vi "HitrapGUI.HTLE_TR6BT1-copy.vi"() -> ()   [LabVIEW 2014, in "HT_CSGUI.lvlib"]
uses:
  HT_CSGUI.lvlib
  CSlibraries/UtilityLib/UtilityLib.lvlib
  CSCore/CSSystem/CSSystemLib/CSSystemLib.lvlib
  CSlibraries/GUILib/GUILib.lvlib
  CSlibraries/UtilityLib/UtilityLib.valueStatus.ctl
  CSCore/CSSystem/CoreDefs/CoreDefs.rawDataType.ctl
  CSCore/CSSystem/CoreLib/CoreLib.lvlib
  CSCore/CSSystem/CoreLib/CoreLib.double 2 byte array.vi
  CSlibraries/GUILib/GUILib.userEventsMainType.ctl
  lib.lib/DimLVEvent/DimIndicators/DimIndicators.anyType.ctl
  CSlibraries/GUILib/GUILib.simpleNumeric.ctl
  CSlibraries/GUILib/GUILib.basicNumeric.ctl
panel:
  in  "showHigh":bool=TRUE
  in  "TR6BT1Trap17_H":bool=TRUE
  in  "TR6BT1Trap16_H":bool=TRUE
  in  "TR6BT1Trap15_H":bool=TRUE
  in  "TR6BT1Trap14_H":bool=TRUE
  in  "TR6BT1Trap13_H":bool=TRUE
  in  "TR6BT1Trap12_H":bool=TRUE
  in  "TR6BT1Trap8_H":bool=TRUE
  in  "TR6BT1Trap7_H":bool=TRUE
  in  "TR6BT1Trap5_H":bool=TRUE
  in  "TR6BT1Trap4_H":bool=TRUE
  in  "TR6BT1Trap3_H":bool=TRUE
  in  "TR6BT1Trap2_H":bool=TRUE
  in  "TR6BT1Trap21_H":bool=TRUE
  in  "TR6BT1Trap20_H":bool=TRUE
  in  "TR6BT1Trap19_H":bool=TRUE
  in  "TR6BT1Trap18_H":bool=TRUE
  in  "TR6BT1Trap11_H":bool=TRUE
  in  "TR6BT1Trap10_H":bool=TRUE
  in  "TR6BT1Trap9_H":bool=TRUE
  in  "TR6BT1Trap6_H":bool=TRUE
  in  "TR6BT1Trap1_H":bool=TRUE
  in  "TR6BT1Trap2":bool=TRUE
  in  "TR6BT1Trap21":bool=TRUE
  in  "TR6BT1Trap20":bool=TRUE
  in  "TR6BT1Trap19":bool=TRUE
  in  "TR6BT1Trap18":bool=TRUE
  in  "TR6BT1Trap17":bool=TRUE
  in  "TR6BT1Trap16":bool=TRUE
  in  "TR6BT1Trap15":bool=TRUE
  in  "TR6BT1Trap14":bool=TRUE
  in  "TR6BT1Trap13":bool=TRUE
  in  "TR6BT1Trap12":bool=TRUE
  in  "TR6BT1Trap11":bool=TRUE
  in  "TR6BT1Trap10":bool=TRUE
  in  "TR6BT1Trap9":bool=TRUE
  in  "TR6BT1Trap8":bool=TRUE
  in  "TR6BT1Trap7":bool=TRUE
  in  "TR6BT1Trap6":bool=TRUE
  in  "TR6BT1Trap5":bool=TRUE
  in  "TR6BT1Trap4":bool=TRUE
  in  "TR6BT1Trap3":bool=TRUE
  in  "TR6BT1Trap11_HCtl":T1 {"nom" step=1.0}
  in  "TR6BT1Trap11Ctl":T1 {"nom" step=1.0}
  in  "TR6BT1Trap10Ctl":T1 {"nom" step=1.0}
  in  "TR6BT1Trap10_HCtl":T1 {"nom" step=1.0}
  in  "TR6BT1Trap9Ctl":T1 {"nom" step=1.0}
  in  "TR6BT1Trap4_HCtl":T1 {"nom" step=1.0}
  in  "TR6BT1Trap9_HCtl":T1 {"nom" step=1.0}
  in  "TR6BT1Trap12_HCtl":T1 {"nom" step=1.0}
  in  "TR6BT1Trap21_HCtl":T1 {"nom" step=1.0}
  in  "TR6BT1Trap8_HCtl":T1 {"nom" step=1.0}
  in  "TR6BT1Trap7_HCtl":T1 {"nom" step=1.0}
  in  "TR6BT1Trap7Ctl":T1 {"nom" step=1.0}
  in  "TR6BT1Trap5Ctl":T1 {"nom" step=1.0}
  in  "TR6BT1Trap12Ctl":T1 {"nom" step=1.0}
  in  "TR6BT1Trap21Ctl":T1 {"nom" step=1.0}
  in  "TR6BT1Trap8Ctl":T1 {"nom" step=1.0}
  in  "TR6BT1Trap6Ctl":T1 {"nom" step=1.0}
  in  "TR6BT1Trap6_HCtl":T1 {"nom" step=1.0}
  in  "TR6BT1Trap5_HCtl":T1 {"nom" step=1.0}
  in  "TR6BT1Trap4Ctl":T1 {"nom" step=1.0}
  in  "TR6BT1Trap3_HCtl":T1 {"nom" step=1.0}
  in  "TR6BT1Trap2Ctl":T1 {"nom" step=1.0}
  in  "TR6BT1Trap3Ctl":T1 {"nom" step=1.0}
  in  "TR6BT1Trap2_HCtl":T1 {"nom" step=1.0}
  in  "TR6BT1Trap19Ctl":T1 {"nom" step=1.0}
  in  "TR6BT1Trap20_HCtl":T1 {"nom" step=1.0}
  in  "TR6BT1Trap17_HCtl":T1 {"nom" step=1.0}
  in  "TR6BT1Trap18_HCtl":T1 {"nom" step=1.0}
  in  "TR6BT1Trap20Ctl":T1 {"nom" step=1.0}
  in  "TR6BT1Trap19_HCtl":T1 {"nom" step=1.0}
  in  "TR6BT1Trap18Ctl":T1 {"nom" step=1.0}
  in  "TR6BT1Trap17Ctl":T1 {"nom" step=1.0}
  in  "TR6BT1Trap16Ctl":T1 {"nom" step=1.0}
  in  "TR6BT1Trap15Ctl":T1 {"nom" step=1.0}
  in  "TR6BT1Trap16_HCtl":T1 {"nom" step=1.0}
  in  "TR6BT1Trap15_HCtl":T1 {"nom" step=1.0}
  in  "TR6BT1Trap14Ctl":T1 {"nom" step=1.0}
  in  "TR6BT1Trap14_HCtl":T1 {"nom" step=1.0}
  in  "TR6BT1Trap13Ctl":T1 {"nom" step=1.0}
  in  "TR6BT1Trap13_HCtl":T1 {"nom" step=1.0}
  in  "TR6BT1Trap1_HCtl":T1 {"nom" step=1.0}
  in  "OK Button":bool
  in  "TR6BT1Trap1Ctl":T1 {"nom" step=1.0}
  in  "TR6BT1Trap1":bool=TRUE
  in  "analog1Ctl":T1 {"nom" step=1.0}
  in  "analog1":bool=TRUE
  out "subSystem1State":string
  in  "subSystem1":bool
  out "subSystem1StateQuality":string
  in  "subControllersIgnoredDIM":T3
  in  "iniData":string
  in  "stop":bool
  in  "dummy":bool
  in  "parentSystem":bool
  in  "userEvent":refnum<user-event>
  # "TR6BT1"
  # "1"
  # "2"
  # "3"
  # "4"
  # "5"
  # "6"
  # "7"
  # "8"
  # "9"
  # "10"
  # "11"
  # "12"
  # "13"
  # "14"
  # "15"
  # "16"
  # "17"
  # "18"
  # "19"
  # "20"
  # "21"
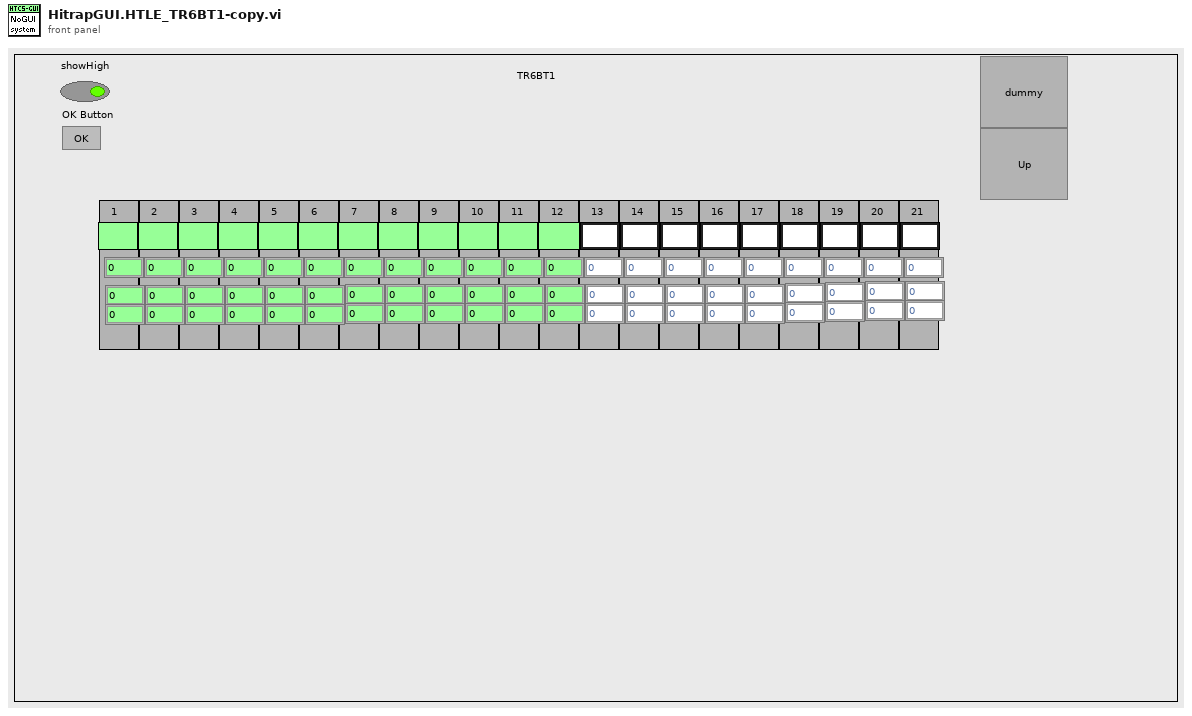
[diagram p1: front panel]
types:
  T1 = typedef "GUILib.lvlib/GUILib.simpleNumeric.ctl" = cluster{"nom":T2, "act":dbl, "inc":dbl}
  T2 = typedef "GUILib.lvlib/GUILib.basicNumeric.ctl" = dbl
  T3 = typedef "DimIndicators.lvlib/DimIndicators.anyType.ctl" = cluster{"data":string, "no link":bool, "quality":i32, "timeStamp":dbl}
  T4 = typedef "UtilityLib.lvlib/UtilityLib.valueStatus.ctl" = enum16{"no info available", "stand by/off", "on", "warning", "alarm/malfunction", "not implemented", "user action required", "important information", "system default", "control default", "indicator default", "button default"}
  T5 = typedef "CoreDefs.rawDataType.ctl" = i8[]
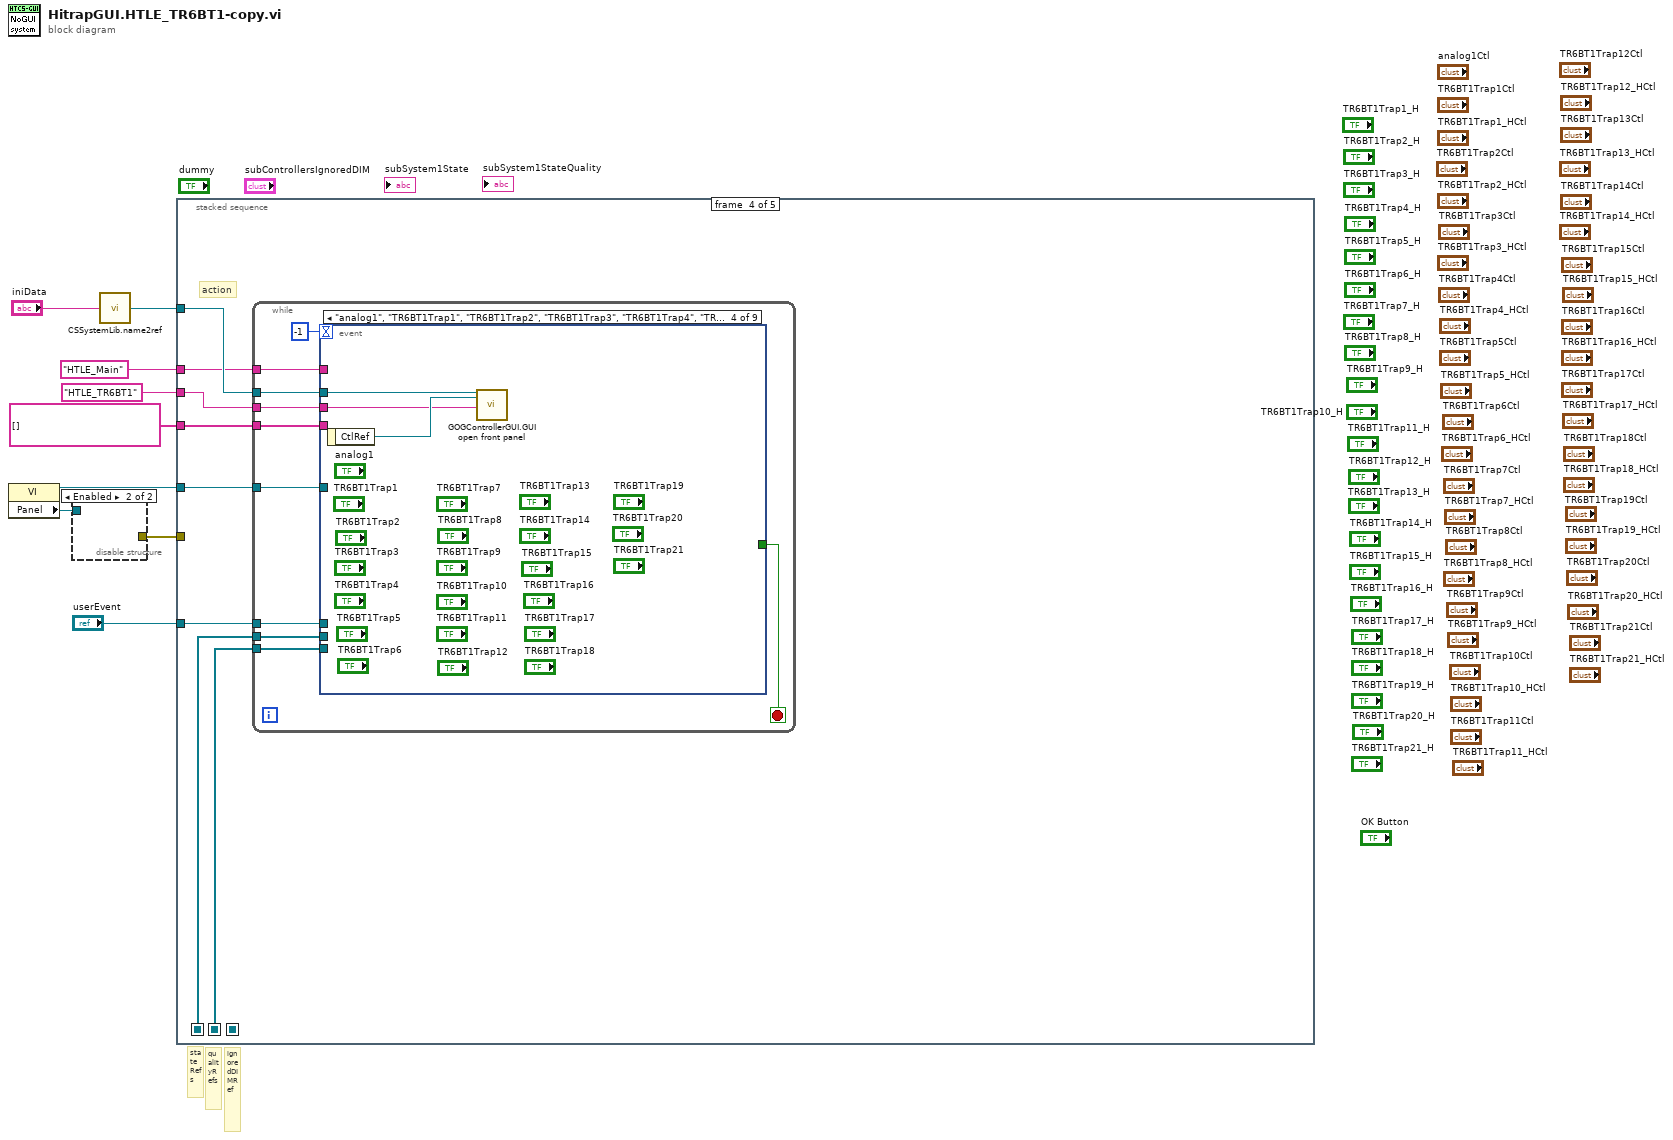
[diagram p0: block diagram]
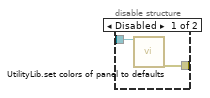
[diagram p2: hidden frame]
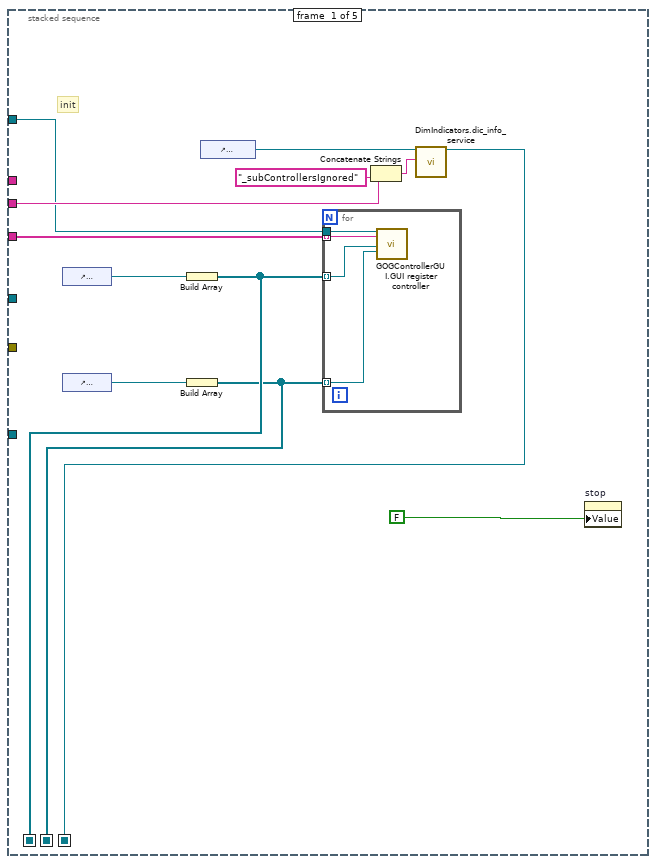
[diagram p3: hidden frame]
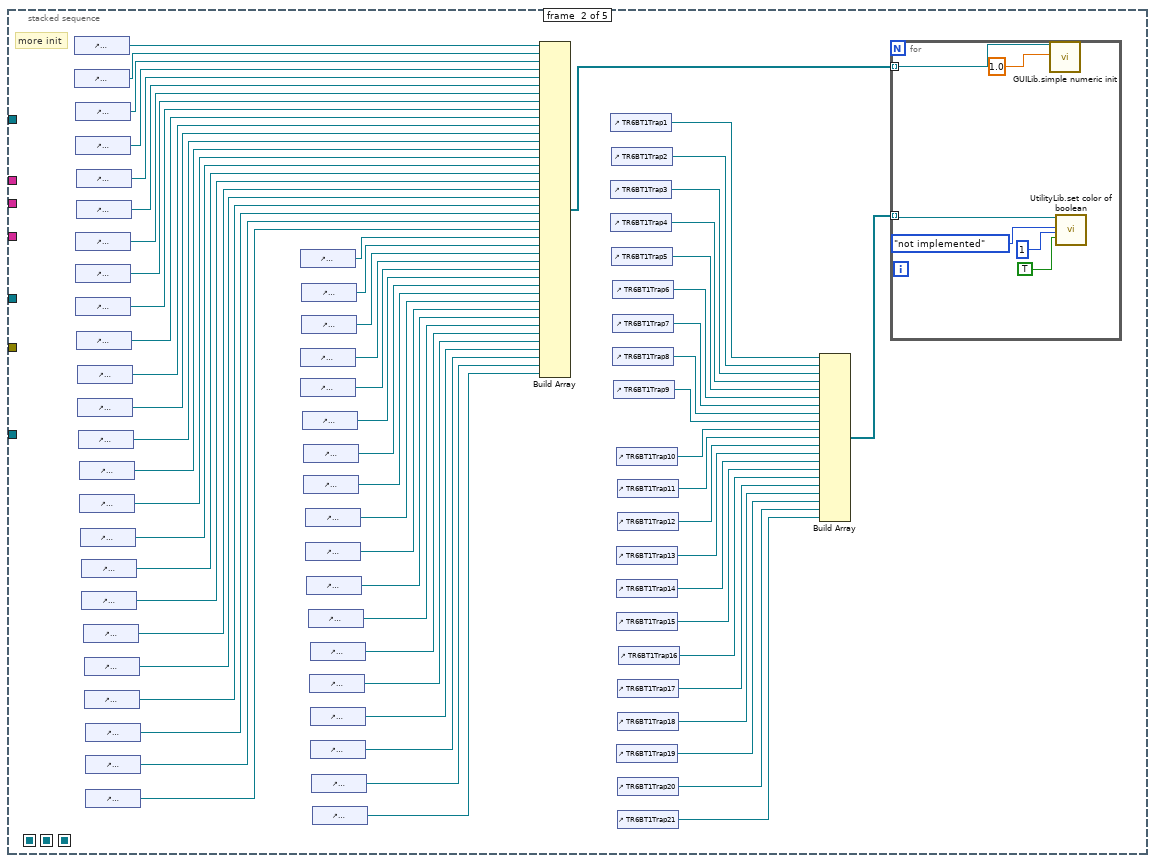
[diagram p4: hidden frame]
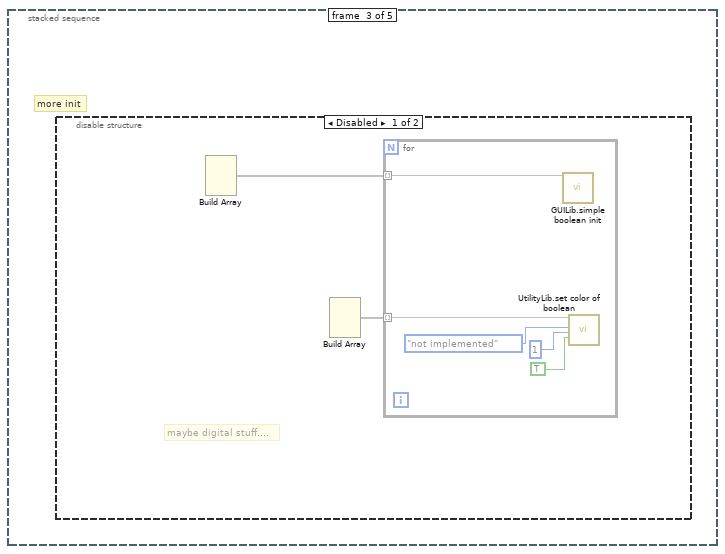
[diagram p5: hidden frame]
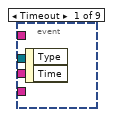
[diagram p7: hidden frame]
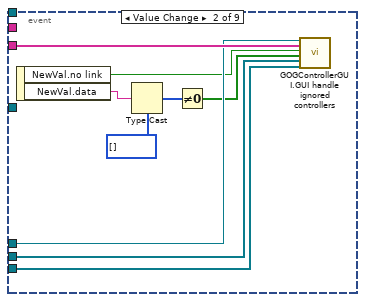
[diagram p8: hidden frame]
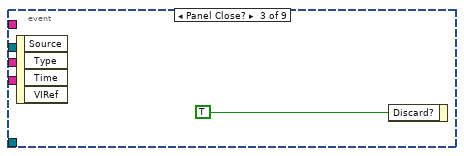
[diagram p9: hidden frame]
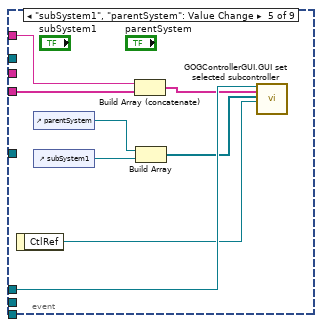
[diagram p10: hidden frame]
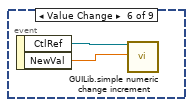
[diagram p11: hidden frame]
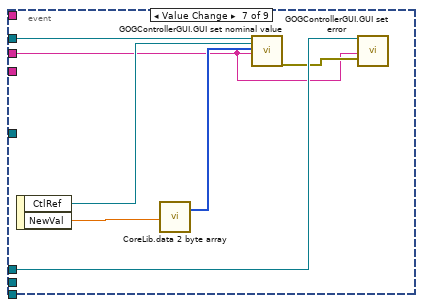
[diagram p12: hidden frame]
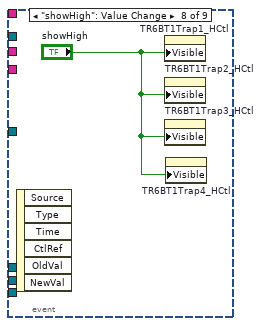
[diagram p13: hidden frame]
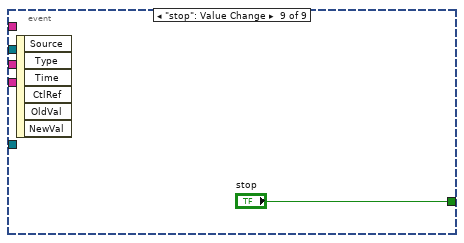
[diagram p14: hidden frame]
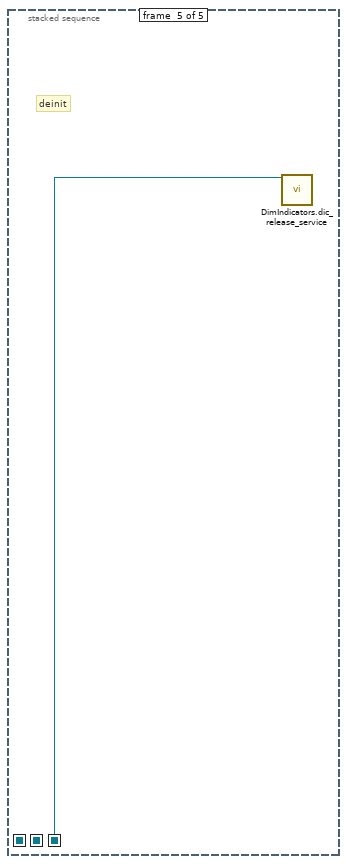
[diagram p15: hidden frame]
diagram:
  # "qualityRefs"
  # "ignoredDIMRef"
  # "stateRefs"
  n1 = property class="VI"() -> (reference out=w7:refnum<vi>, "Panel"=w8:refnum<vi>)  [unwired: 2 in, 1 out]
  n2 = disable-structure shown="Enabled" {
    disable-tunnel: w8 -> [w11 _]
    disable-tunnel: [w10 _] -> w6
    frame Disabled {
      n3 = call "UtilityLib.set colors of panel to defaults.vi"("Front Panel"=w11) -> ("error out"=w10:errorcluster)  [unwired: 18 in]
    }
    frame Enabled {
    }
  }
  n4 = call "CSSystemLib.name2ref.vi"("name"="iniData") -> ("obj refnum"=w2:refnum<vi>)
  n5 = stacked-sequence {
    seq-local: [w13 _ _ _ _] -> [_ _ _ _ w166]
    seq-local: [w14 _ _ _ _] -> [_ _ _ w120 _]
    seq-local: [w12 _ _ _ _] -> [_ _ _ w119 _]
    tunnel: "userEvent" -> [_ _ _ w123 _]
    tunnel: w7 -> [_ _ _ w122 _]
    tunnel: w6 -> [_ _ _ _ _]
    tunnel: "HTLE_TR6BT1" -> [w19 _ _ w117 _]
    tunnel: string[] [] -> [w18 _ _ w121 _]
    tunnel: w2 -> [w17 _ _ w118 _]
    tunnel: "HTLE_Main" -> [_ _ _ w116 _]
    frame #0 {
      # "init"
      n6 = control-ref of="dummySubSystemState"() -> (w16:refnum<vi>)
      n7 = control-ref of="dummySubSystemStateQuality"() -> (w15:refnum<vi>)
      n8 = Build Array(w16) -> (w14:refnum<vi>[])
      n9 = Build Array(w15) -> (w12:refnum<vi>[])
      n10 = control-ref of="subControllersIgnoredDIM"() -> (w20:refnum<vi>)
      n11 = for {
        tunnel: w14 -> [w27] mode=indexing
        tunnel: w18 -> [w25] mode=indexing
        tunnel: w12 -> [w24] mode=indexing
        tunnel: w17 -> [w26]
        n12 = call "GOGControllerGUI.GUI register controller.vi"("i ref in"=w26, "controllerName"=w25, "subSystemState"=w27, "subSystemStateQuality"=w24) -> ()  [unwired: 14 in, 2 out]
      }
      n13 = Concatenate Strings(w19, "_subControllersIgnored" ("string")) -> (w22:string)
      n14 = call "DimIndicators.dic_info_service.vi"("controlRef"=w20, "serviceName"=w22) -> ("controlRef out"=w13:refnum<vi>)  [unwired: 16 in, 1 out]
      n15 = property on="stop" class="Bool (strict)"("Value"=FALSE ("stop")) -> ()  [unwired: 2 in, 2 out]
    }
    frame #1 {
      # "more init"
      n16 = control-ref of="TR6BT1Trap1Ctl"() -> (w92:refnum<vi>)
      n17 = control-ref of="TR6BT1Trap1_HCtl"() -> (w88:refnum<vi>)
      n18 = control-ref of="TR6BT1Trap2Ctl"() -> (w87:refnum<vi>)
      n19 = control-ref of="TR6BT1Trap2_HCtl"() -> (w86:refnum<vi>)
      n20 = control-ref of="TR6BT1Trap4Ctl"() -> (w83:refnum<vi>)
      n21 = control-ref of="TR6BT1Trap4_HCtl"() -> (w82:refnum<vi>)
      n22 = control-ref of="TR6BT1Trap5Ctl"() -> (w81:refnum<vi>)
      n23 = control-ref of="TR6BT1Trap3Ctl"() -> (w85:refnum<vi>)
      n24 = control-ref of="TR6BT1Trap3_HCtl"() -> (w84:refnum<vi>)
      n25 = control-ref of="TR6BT1Trap5_HCtl"() -> (w80:refnum<vi>)
      n26 = control-ref of="TR6BT1Trap6Ctl"() -> (w79:refnum<vi>)
      n27 = control-ref of="TR6BT1Trap6_HCtl"() -> (w78:refnum<vi>)
      n28 = control-ref of="TR6BT1Trap7Ctl"() -> (w77:refnum<vi>)
      n29 = control-ref of="TR6BT1Trap7_HCtl"() -> (w76:refnum<vi>)
      n30 = control-ref of="TR6BT1Trap8Ctl"() -> (w75:refnum<vi>)
      n31 = control-ref of="TR6BT1Trap8_HCtl"() -> (w74:refnum<vi>)
      n32 = control-ref of="TR6BT1Trap9Ctl"() -> (w73:refnum<vi>)
      n33 = control-ref of="TR6BT1Trap9_HCtl"() -> (w72:refnum<vi>)
      n34 = control-ref of="TR6BT1Trap10Ctl"() -> (w70:refnum<vi>)
      n35 = control-ref of="TR6BT1Trap10_HCtl"() -> (w69:refnum<vi>)
      n36 = control-ref of="TR6BT1Trap11Ctl"() -> (w68:refnum<vi>)
      n37 = control-ref of="TR6BT1Trap11_HCtl"() -> (w67:refnum<vi>)
      n38 = control-ref of="TR6BT1Trap12Ctl"() -> (w66:refnum<vi>)
      n39 = control-ref of="TR6BT1Trap12_HCtl"() -> (w65:refnum<vi>)
      n40 = control-ref of="TR6BT1Trap13Ctl"() -> (w64:refnum<vi>)
      n41 = control-ref of="TR6BT1Trap14_HCtl"() -> (w61:refnum<vi>)
      n42 = control-ref of="TR6BT1Trap15Ctl"() -> (w60:refnum<vi>)
      n43 = control-ref of="TR6BT1Trap13_HCtl"() -> (w63:refnum<vi>)
      n44 = control-ref of="TR6BT1Trap14Ctl"() -> (w62:refnum<vi>)
      n45 = control-ref of="TR6BT1Trap15_HCtl"() -> (w59:refnum<vi>)
      n46 = control-ref of="TR6BT1Trap16Ctl"() -> (w58:refnum<vi>)
      n47 = control-ref of="TR6BT1Trap16_HCtl"() -> (w57:refnum<vi>)
      n48 = control-ref of="TR6BT1Trap17Ctl"() -> (w56:refnum<vi>)
      n49 = control-ref of="TR6BT1Trap17_HCtl"() -> (w55:refnum<vi>)
      n50 = control-ref of="TR6BT1Trap18Ctl"() -> (w54:refnum<vi>)
      n51 = control-ref of="TR6BT1Trap18_HCtl"() -> (w53:refnum<vi>)
      n52 = control-ref of="TR6BT1Trap19_HCtl"() -> (w51:refnum<vi>)
      n53 = control-ref of="TR6BT1Trap19Ctl"() -> (w52:refnum<vi>)
      n54 = control-ref of="TR6BT1Trap20Ctl"() -> (w50:refnum<vi>)
      n55 = control-ref of="TR6BT1Trap20_HCtl"() -> (w49:refnum<vi>)
      n56 = control-ref of="TR6BT1Trap21Ctl"() -> (w48:refnum<vi>)
      n57 = control-ref of="TR6BT1Trap21_HCtl"() -> (w47:refnum<vi>)
      n58 = Build Array(w92, w88, w87, w86, w85, w84, w83, w82, w81, w80, w79, w78, w77, w76, w75, w74, w73, w72, w70, w69, w68, w67, w66, w65, w64, w63, w62, w61, w60, w59, w58, w57, w56, w55, w54, w53, w52, w51, w50, w49, w48, w47) -> (w91:refnum<vi>[])
      n59 = control-ref of="TR6BT1Trap1"() -> (w90:refnum<vi>)
      n60 = control-ref of="TR6BT1Trap3"() -> (w46:refnum<vi>)
      n61 = control-ref of="TR6BT1Trap4"() -> (w45:refnum<vi>)
      n62 = control-ref of="TR6BT1Trap2"() -> (w71:refnum<vi>)
      n63 = control-ref of="TR6BT1Trap5"() -> (w44:refnum<vi>)
      n64 = control-ref of="TR6BT1Trap6"() -> (w43:refnum<vi>)
      n65 = control-ref of="TR6BT1Trap7"() -> (w42:refnum<vi>)
      n66 = control-ref of="TR6BT1Trap8"() -> (w41:refnum<vi>)
      n67 = control-ref of="TR6BT1Trap9"() -> (w40:refnum<vi>)
      n68 = control-ref of="TR6BT1Trap10"() -> (w39:refnum<vi>)
      n69 = control-ref of="TR6BT1Trap13"() -> (w36:refnum<vi>)
      n70 = control-ref of="TR6BT1Trap14"() -> (w35:refnum<vi>)
      n71 = control-ref of="TR6BT1Trap15"() -> (w34:refnum<vi>)
      n72 = control-ref of="TR6BT1Trap19"() -> (w30:refnum<vi>)
      n73 = control-ref of="TR6BT1Trap11"() -> (w38:refnum<vi>)
      n74 = control-ref of="TR6BT1Trap12"() -> (w37:refnum<vi>)
      n75 = control-ref of="TR6BT1Trap17"() -> (w32:refnum<vi>)
      n76 = control-ref of="TR6BT1Trap18"() -> (w31:refnum<vi>)
      n77 = control-ref of="TR6BT1Trap20"() -> (w29:refnum<vi>)
      n78 = control-ref of="TR6BT1Trap21"() -> (w28:refnum<vi>)
      n79 = control-ref of="TR6BT1Trap16"() -> (w33:refnum<vi>)
      n80 = Build Array(w90, w71, w46, w45, w44, w43, w42, w41, w40, w39, w38, w37, w36, w35, w34, w33, w32, w31, w30, w29, w28) -> (w89:refnum<vi>[])
      n81 = for {
        tunnel: w91 -> [w98] mode=indexing
        tunnel: w89 -> [w94] mode=indexing
        n82 = call "GUILib.simple numeric init.vi"("ctlRef"=w98, "increment"=1.0) -> ()  [unwired: 16 in, 2 out]
        n83 = call "UtilityLib.set color of boolean.vi"("button"=w94, "valueStatus"=UtilityLib.valueStatus."not implemented", "nOfPair (0)"=1, "setTRUEColor (FALSE)"=TRUE) -> ()  [unwired: 15 in, 1 out]
      }
    }
    frame #2 {
      # "more init"
      n84 = disable-structure shown="Disabled" {
        frame Disabled {
          # "maybe digital stuff...."
          n85 = Build Array() -> (w105:void[], w110:dbl, w109:dbl, w108:dbl, w107:dbl, w106:dbl)
          n86 = Build Array() -> (w99:void[], w104:dbl, w103:dbl, w102:dbl, w101:dbl, w100:dbl)
          n87 = for {
            tunnel: w105 -> [w115] mode=indexing
            tunnel: w99 -> [w111] mode=indexing
            n88 = call "GUILib.simple boolean init.vi"("ctlRef"=w115) -> ()  [unwired: 17 in, 2 out]
            n89 = call "UtilityLib.set color of boolean.vi"("button"=w111, "valueStatus"=UtilityLib.valueStatus."not implemented", "nOfPair (0)"=1, "setTRUEColor (FALSE)"=TRUE) -> ()  [unwired: 15 in, 1 out]
          }
        }
        frame Enabled {
        }
      }
    }
    frame #3 {
      # "action"
      n90 = while {
        tunnel: w123 -> [w133]
        tunnel: w122 -> [w131]
        tunnel: w121 -> [w129]
        tunnel: w120 -> [w128]
        tunnel: w119 -> [w127]
        tunnel: w118 -> [w126]
        tunnel: w117 -> [w125]
        tunnel: w116 -> [w124]
        stop <- w130 stop-if-true
        n91 = event shown="[3] \"analog1\", \"TR6BT1Trap1\", \"TR6BT1Trap2\", \"TR6BT1Trap3\", \"TR6BT1Trap4\", \"TR6BT1Trap5\", \"TR6BT1Trap6\", \"TR6BT1Trap7\", \"TR6BT1Trap8\", \"TR6BT1Trap9\", \"TR6BT1Trap10\", \"TR6BT1Trap11\", \"TR6BT1Trap12\", \"TR6BT1Trap13\", \"TR6BT1Trap14\", \"TR6BT1Trap15\", \"TR6BT1Trap16\", \"TR6BT1Trap17\", \"TR6BT1Trap18\", \"TR6BT1Trap19\", \"TR6BT1Trap20\", \"TR6BT1Trap21\": Value Change" {
          selector: _ -> [_ _ _ _ _ _ _ _ _]
          dyn-events: _ -> [_ _ _ _ _ _ _ _ _]
          timeout: -1 -> [_ _ _ _ _ _ _ _ _]
          tunnel: w133 -> [_ w138 _ _ w153 _ w159 _ _]
          tunnel: w131 -> [_ _ _ _ _ _ _ _ _]
          tunnel: [_ _ _ _ _ _ _ _ "stop"] -> w130
          tunnel: w129 -> [_ w139 _ _ w149 _ _ _ _]
          tunnel: w128 -> [_ w135 _ _ _ _ _ _ _]
          tunnel: w127 -> [_ w134 _ _ _ _ _ _ _]
          tunnel: w126 -> [_ _ _ w146 _ _ w163 _ _]
          tunnel: w125 -> [_ _ _ w144 _ _ w157 _ _]
          tunnel: w124 -> [_ _ _ _ w148 _ _ _ _]
          event Timeout {
            n92 = event-data() -> ()  [unwired: 1 in, 2 out]
          }
          event Value Change {
            n93 = event-data() -> ("NewVal.no link"=w137:bool, "NewVal.data"=w140:string)  [unwired: 1 in]
            n94 = Type Cast(type=T5 [] ("Array"), x=w140) -> (*(type *) &x=w142:T5)
            n95 = Not Equal To 0?(x=w142) -> (x != 0?=w136:bool[])
            n96 = call "GOGControllerGUI.GUI handle ignored controllers.vi"("userEvent"=w138, "controllerNames"=w139, "NOLINK"=w137, "controllersIgnored"=w136, "stateRefs"=w135, "qualityRefs"=w134) -> ()  [unwired: 14 in]
          }
          event Panel Close? {
            n97 = event-data() -> ()  [unwired: 1 in, 4 out]
            n98 = event-data("Discard?"=TRUE) -> ()  [unwired: 1 in, 1 out]
          }
          event "analog1", "TR6BT1Trap1", "TR6BT1Trap2", "TR6BT1Trap3", "TR6BT1Trap4", "TR6BT1Trap5", "TR6BT1Trap6", "TR6BT1Trap7", "TR6BT1Trap8", "TR6BT1Trap9", "TR6BT1Trap10", "TR6BT1Trap11", "TR6BT1Trap12", "TR6BT1Trap13", "TR6BT1Trap14", "TR6BT1Trap15", "TR6BT1Trap16", "TR6BT1Trap17", "TR6BT1Trap18", "TR6BT1Trap19", "TR6BT1Trap20", "TR6BT1Trap21": Value Change {
            n99 = event-data() -> ("CtlRef"=w145:refnum<vi>)  [unwired: 1 in]
            n100 = call "GOGControllerGUI.GUI open front panel.vi"("i ref in"=w146, "elementRef"=w145, "controller"=w144) -> ()  [unwired: 15 in, 2 out]
          }
          event "subSystem1", "parentSystem": Value Change {
            n101 = event-data() -> ("CtlRef"=w151:refnum<vi>)  [unwired: 1 in]
            n102 = control-ref of="parentSystem"() -> (w150:refnum<vi>)
            n103 = control-ref of="subSystem1"() -> (w154:refnum<vi>)
            n104 = Build Array (concatenate)(w148, w149) -> (w147:string[])
            n105 = Build Array(w150, w154) -> (w152:refnum<vi>[])
            n106 = call "GOGControllerGUI.GUI set selected subcontroller.vi"("userEvent"=w153, "controllerNames"=w147, "controllerRefs"=w152, "controllerRef"=w151) -> ()  [unwired: 16 in]
          }
          event Value Change {
            n107 = event-data() -> ("CtlRef"=w156:refnum<vi>, "NewVal"=w155:dbl)  [unwired: 1 in]
            n108 = call "GUILib.simple numeric change increment.vi"("ctlRef"=w156, "increment"=w155) -> ()  [unwired: 16 in, 2 out]
          }
          event Value Change {
            n109 = event-data() -> ("CtlRef"=w162:refnum<vi>, "NewVal"=w161:T2)  [unwired: 1 in]
            n110 = call-poly "CoreLib.data 2 byte array.vi"("f64"=w161) -> ("byteArray out"=w160:T5)  [unwired: 18 in]
            n111 = call "GOGControllerGUI.GUI set nominal value.vi"("i ref in"=w163, "nominalRef"=w162, "nominalData"=w160, "controller"=w157) -> ("error out"=w158:errorcluster)  [unwired: 14 in, 1 out]
            n112 = call "GOGControllerGUI.GUI set error.vi"("userEvent"=w159, "controller"=w157, "GUIError"=w158) -> ()  [unwired: 16 in, 1 out]
          }
          event "showHigh": Value Change {
            n113 = event-data() -> ()  [unwired: 1 in, 6 out]
            n114 = property on="TR6BT1Trap1_HCtl" class="Clust (strict)"("Visible"="showHigh") -> ()  [unwired: 2 in, 2 out]
            n115 = property on="TR6BT1Trap2_HCtl" class="Clust (strict)"("Visible"="showHigh") -> ()  [unwired: 2 in, 2 out]
            n116 = property on="TR6BT1Trap3_HCtl" class="Clust (strict)"("Visible"="showHigh") -> ()  [unwired: 2 in, 2 out]
            n117 = property on="TR6BT1Trap4_HCtl" class="Clust (strict)"("Visible"="showHigh") -> ()  [unwired: 2 in, 2 out]
          }
          event "stop": Value Change {
            n118 = event-data() -> ()  [unwired: 1 in, 6 out]
          }
        }
      }
    }
    frame #4 {
      # "deinit"
      n119 = call "DimIndicators.dic_release_service.vi"("controlRef"=w166) -> ()  [unwired: 18 in, 1 out]
    }
  }
